vi "Tenma 72-2535 VI Tree.vi"   [LabVIEW 2015]
doc: "VI Tree für die CX (Twincat) Ansteuerung."
uses:
  Tenma 72-2535.llb/72-2535 FunktionValues.ctl
  Tenma 72-2535.lvlib
panel:
  # "SEE DIAGRAM\nFOR VI TREE."
types:
  T1 = typedef "Tenma 72-2535.lvlib/72-2535 FunktionValues.ctl" = enum16{"Voltage Set Write", "Voltage Set Read", "Voltage Out Read", "Current Set Write", "Current Set Read", "Current Out Read"}
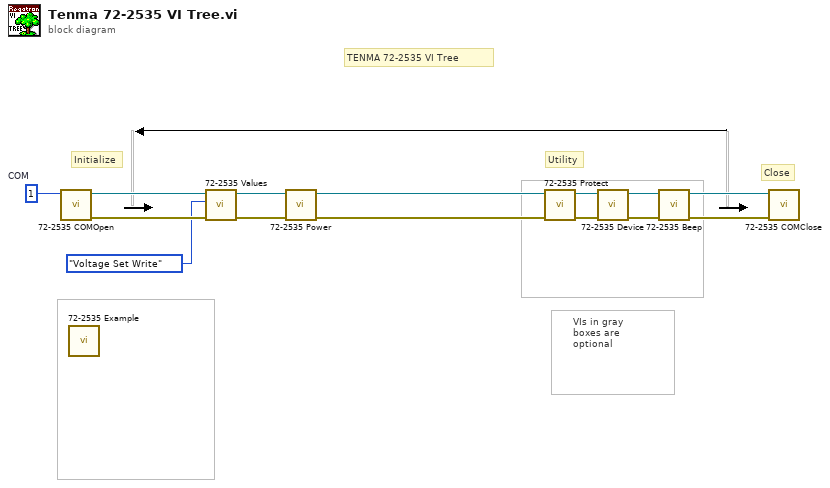
[diagram p0: block diagram]
diagram:
  w14 = u8 1  # COM
  # "VIs in gray\nboxes are\noptional"
  # "TENMA 72-2535 VI Tree"
  # "Utility"
  # "Close"
  # "Initialize"
  n1 = call "72-2535 COMOpen.vi"("COM Port"=w14) -> ("Fehler (Ausgang)"=w13:errorcluster, "VISA-Referenz (Ausgang)"=w12:refnum<visa-resource-name>)  [unwired: 9 in]
  n2 = call "72-2535 Example.vi"() -> ()  [unwired: 11 in, 1 out]
  n3 = call "72-2535 Values.vi"("Fehler (Eingang, kein Fehler)"=w13, "Funktion Values"=72-2535_FunktionValues."Voltage Set Write", "VISA-Referenz (Eingang)"=w12) -> ("Fehler (Ausgang)"=w11:errorcluster, "VISA-Referenz (Ausgang)"=w10:refnum<visa-resource-name>)  [unwired: 6 in, 1 out]
  n4 = call "72-2535 Power.vi"("Fehler (Eingang, kein Fehler)"=w11, "VISA-Referenz (Eingang)"=w10) -> ("Fehler (Ausgang)"=w8:errorcluster, "VISA-Referenz (Ausgang)"=w7:refnum<visa-resource-name>)  [unwired: 8 in]
  n5 = call "72-2535 Protect.vi"("Fehler (Eingang, kein Fehler)"=w8, "VISA-Referenz (Eingang)"=w7) -> ("Fehler (Ausgang)"=w9:errorcluster, "VISA-Referenz (Ausgang)"=w6:refnum<visa-resource-name>)  [unwired: 8 in]
  n6 = call "72-2535 Device.vi"("Fehler (Eingang, kein Fehler)"=w9, "VISA-Referenz (Eingang)"=w6) -> ("Fehler (Ausgang)"=w4:errorcluster, "VISA-Referenz (Ausgang)"=w1:refnum<visa-resource-name>)  [unwired: 6 in, 2 out]
  n7 = call "72-2535 Beep.vi"("Fehler (Eingang, kein Fehler)"=w4, "VISA-Referenz (Eingang)"=w1) -> ("Fehler (Ausgang)"=w3:errorcluster, "VISA-Referenz (Ausgang)"=w2:refnum<visa-resource-name>)  [unwired: 8 in]
  n8 = call "72-2535 COMClose.vi"("Fehler (Eingang, kein Fehler)"=w3, "VISA-Referenz (Eingang)"=w2) -> ()  [unwired: 9 in, 1 out]
